vi "set_params.vi"(8 "error in (no error)":errorcluster caption="entrée d'erreur (pas d'erreur)", 11 "FeatureAgglomeration.lvclass 2":refnum<class "FeatureAgglomeration.lvclass">) -> (0 "error out":errorcluster caption="sortie d'erreur", 3 "FeatureAgglomeration.lvclass":refnum<class "FeatureAgglomeration.lvclass">)   [LabVIEW 2020, in "FeatureAgglomeration.lvclass"]
uses:
  FeatureAgglomeration.lvclass
  FeatureAgglomeration.lvclass/FeatureAgglomeration.ctl
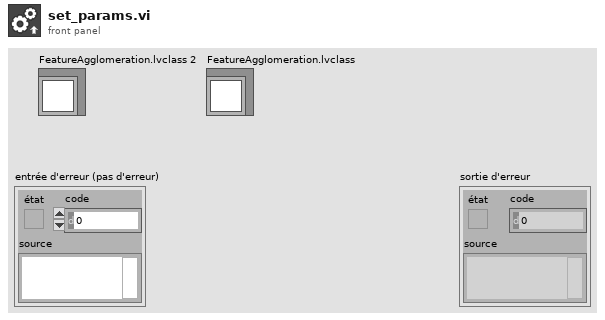
[diagram p1: front panel]
types:
  T1 = typedef "feature_agglomeration_params.ctl" = cluster{"n_clusters":dbl, "affinity":string, "memory":string, "connectivity":cluster{"connectivity_type":string, "connectivity_list":dbl[][]}, "compute_full_tree":cluster{"compute_full_tree_type":string, "compute_full_tree_bool":bool}, "linkage":string, "distance_threshold":cluster{"distance_threshold_type":string, "distance_threshold_float":dbl}, "compute_distances":bool}
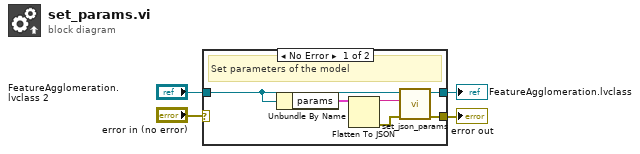
[diagram p0: block diagram]
diagram:
  n1 = case shown="No Error" "error in (no error)" {
    selector: "error in (no error)" -> [_ w12]
    tunnel: [w7 w12] -> w3
    tunnel: [w8 w11] -> w1
    tunnel: "FeatureAgglomeration.lvclass 2" -> [w5 w11]
    frame No Error {
      # "Set parameters of the model"
      n2 = Unbundle By Name(w5) -> ("params"=w10:T1)
      n3 = Flatten To JSON(anything=w10) -> (JSON string=w9:string, 11:w6:errorcluster)  [unwired: 2 in]
      n4 = call-dynamic "set_json_params.vi"("error in (no error)"=w6, "params"=w9, "Model en entrée"=w5) -> ("error out"=w7:errorcluster, "Model en sortie"=w8:refnum<class "FeatureAgglomeration.lvclass">)  [unwired: 7 in]
    }
    frame Error {
    }
  }
  "error out" <- w3
  "FeatureAgglomeration.lvclass" <- w1
